vi "4-6.3.vi"(1 "数值 2":dbl, 2 "数值":dbl) -> (0 "数值 3":dbl)   [LabVIEW 2017]
panel:
  in  "停止":bool
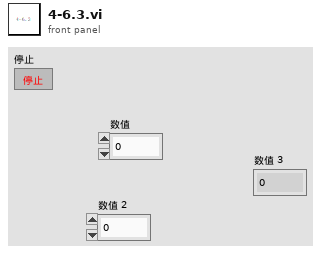
[diagram p1: front panel]
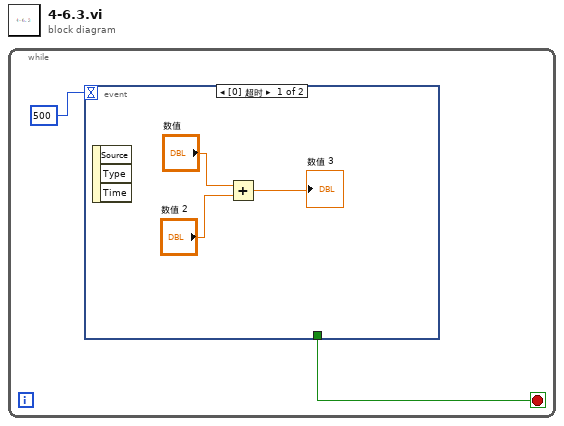
[diagram p0: block diagram]
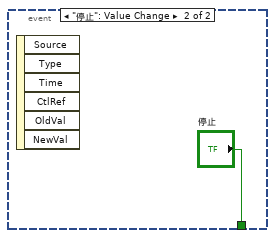
[diagram p2: hidden frame]
diagram:
  n1 = while {
    stop <- w1 stop-if-true
    n2 = event shown="[0] 超时" {
      selector: _ -> [_ _]
      dyn-events: _ -> [_ _]
      timeout: 500 -> [_ _]
      tunnel: [_ "停止"] -> w1
      event Timeout {
        n3 = event-data() -> ()  [unwired: 1 in, 3 out]
        n4 = Add(x="数值", y="数值 2") -> (x+y=→"数值 3":dbl)
      }
      event "停止": Value Change {
        n5 = event-data() -> ()  [unwired: 1 in, 6 out]
      }
    }
  }
